vi "hysteresisCompensation.vi"(8 "error in (no error)":errorcluster, 9 "Polynom":dbl[](array[numeric])=[0.0, 1.0, 0.0, 0.0], 10 "Uncorrected Shape":dbl[](array[numeric])) -> (0 "error out":errorcluster, 2 "Corrected Shape":dbl[](array[numeric]))   [LabVIEW 2016]
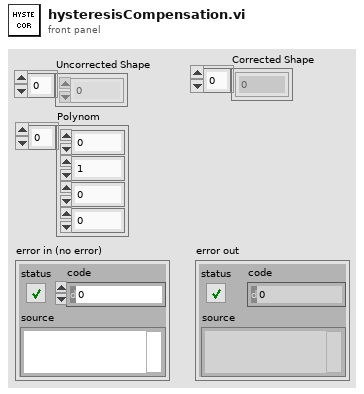
[diagram p1: front panel]
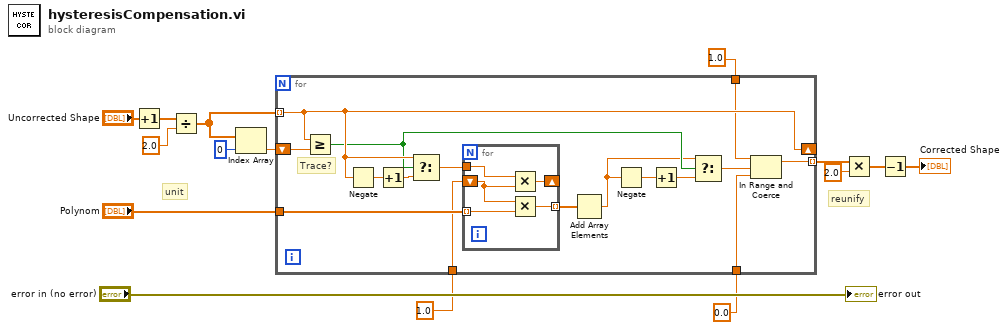
[diagram p0: block diagram]
diagram:
  # "reunify"
  # "unit"
  n1 = Increment(x="Uncorrected Shape") -> (x+1=w1:dbl[])
  n2 = Divide(x=w1, y=2.0) -> (x/y=w7:dbl[])
  n3 = Index Array(array=w7, index=0) -> (element=w14:dbl)
  n4 = for {
    tunnel: w7 -> [w28] mode=indexing
    shift-right: [w28] -> _
    shift-left: w14 -> [w31]
    tunnel: "Polynom" -> [w23]
    tunnel: [w19] -> w12 mode=indexing
    tunnel: 0.0 ("lower limit") -> [w18]
    tunnel: 1.0 ("upper limit") -> [w17]
    tunnel: 1.0 -> [w16]
    # "Trace?"
    n5 = Greater Or Equal?(x=w28, y=w31) -> (x >= y?=w25:bool)
    n6 = Negate(x=w28) -> (-x=w30:dbl)
    n7 = Increment(x=w30) -> (x+1=w29:dbl)
    n8 = Select(t=w28, s=w25, f=w29) -> (s? t:f=w24:dbl)
    n9 = for {
      tunnel: w24 -> [w36]
      tunnel: w23 -> [w33] mode=indexing
      shift-right: [w35] -> _
      shift-left: w16 -> [w34]
      tunnel: [w32] -> w22 mode=indexing
      n10 = Multiply(x=w36, y=w34) -> (x*y=w35:dbl)
      n11 = Multiply(x=w34, y=w33) -> (x*y=w32:dbl)
    }
    n12 = Add Array Elements(numeric array=w22) -> (sum=w21:dbl)
    n13 = Negate(x=w21) -> (-x=w26:dbl)
    n14 = Increment(x=w26) -> (x+1=w27:dbl)
    n15 = Select(t=w21, s=w25, f=w27) -> (s? t:f=w20:dbl)
    n16 = In Range and Coerce(upper limit=w17, x=w20, lower limit=w18) -> (coerced(x)=w19:dbl)  [unwired: 1 out]
  }
  n17 = Multiply(x=w12, y=2.0) -> (x*y=w10:dbl[])
  n18 = Decrement(x=w10) -> (x-1=→"Corrected Shape":dbl[])
  "error out" <- "error in (no error)"
